vi "Find Removed Sections.vi"(9 "Offset":u32, 10 "Reference":string, 11 "Target":string) -> (3 "Sections in Reference":T1(array[cluster]))   [LabVIEW 2020]
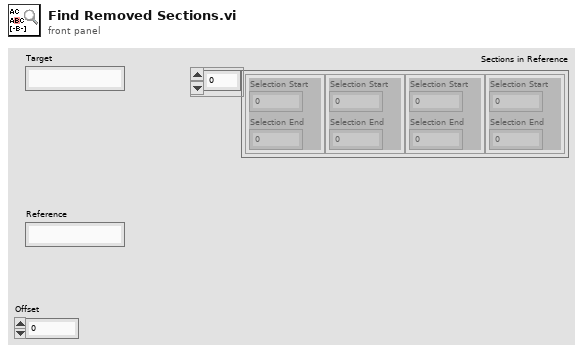
[diagram p1: front panel]
types:
  T1 = cluster{"Selection Start":u32, "Selection End":u32}[]
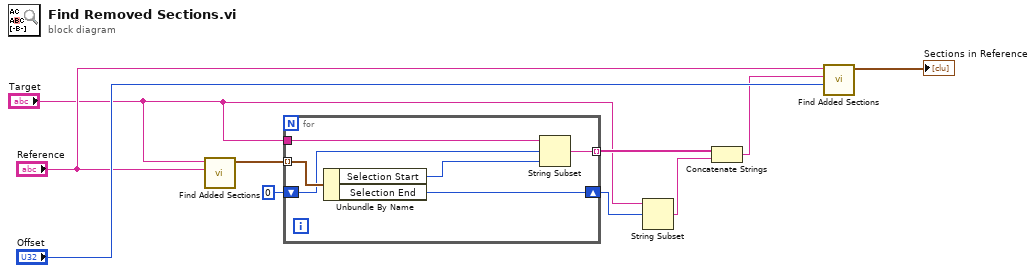
[diagram p0: block diagram]
diagram:
  n1 = call "Find Added Sections.vi"("Reference"="Reference", "Target"="Target") -> ("Sections in Target"=w7:T1)  [unwired: 9 in]
  n2 = for {
    tunnel: w7 -> [w15] mode=indexing
    tunnel: "Target" -> [w16]
    shift-right: [w14] -> w2
    shift-left: u32 0 ("Selection End") -> [w11]
    tunnel: [w13] -> w5 mode=indexing
    n3 = Unbundle By Name(w15) -> ("Selection Start"=w12:u32, "Selection End"=w14:u32)
    n4 = String Subset(string=w16, offset (0)=w11, length (rest)=w12) -> (substring=w13:string)
  }
  n5 = String Subset(string="Target", offset (0)=w2) -> (substring=w1:string)  [unwired: 1 in]
  n6 = Concatenate Strings(w5, w1) -> (w4:string)
  n7 = call "Find Added Sections.vi"("Offset"="Offset", "Reference"=w4, "Target"="Reference") -> ("Sections in Target"=→"Sections in Reference":T1)  [unwired: 8 in]
